vi "Passwort Filter.vi"(9 "Passworte":T1, 10 "aktueller Level":i16) -> (0 "Array Größe":i32, 1 "gefilterte Indexe":i32[](array[numeric]), 2 "Passworte gefiltert":T1)   [LabVIEW 2020, in "Passwort.lvlib"]
uses:
  Passwort.lvlib
  Passwort Array.ctl
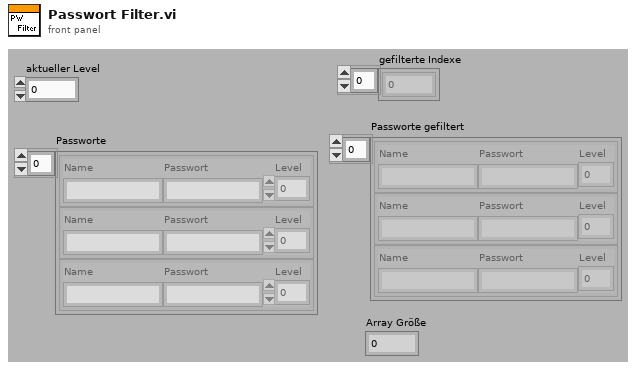
[diagram p1: front panel]
types:
  T1 = typedef "Passwort.lvlib/Passwort Array.ctl" = cluster{"Name":string, "Passwort":string, "Level":i16}[]
  T2 = cluster{"Name":string, "Passwort":string, "Level":i16}
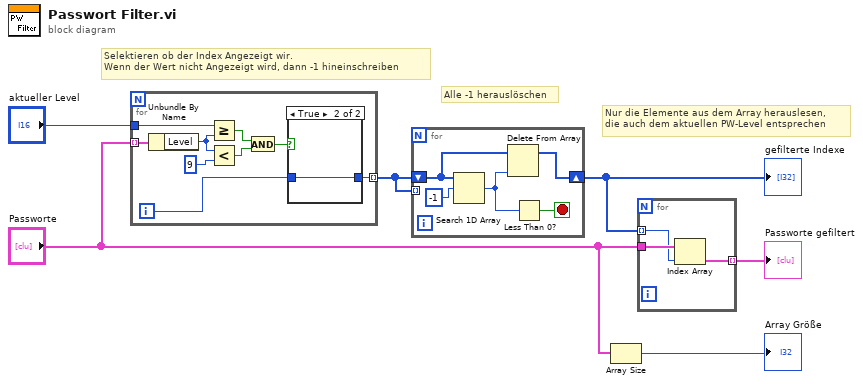
[diagram p0: block diagram]
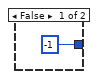
[diagram p2: hidden frame]
diagram:
  # "Nur die Elemente aus dem Array herauslesen, \ndie auch dem aktuellen PW-Level entsprechen"
  # "Alle -1 herauslöschen"
  # "Selektieren ob der Index Angezeigt wir.\nWenn der Wert nicht Angezeigt wird, dann -1 hineinschreiben"
  n1 = for {
    tunnel: "Passworte" -> [w14] mode=indexing
    tunnel: "aktueller Level" -> [w15]
    tunnel: [w12] -> w5 mode=indexing
    i -> [w13]
    n2 = Unbundle By Name(w14) -> ("Level"=w10:i16)
    n3 = Greater Or Equal?(x=w15, y=w10) -> (x >= y?=w8:bool)
    n4 = Less?(x=w10, y=i16 9) -> (x < y?=w11:bool)
    n5 = And(x=w8, y=w11) -> (x .and. y?=w7:bool)
    n6 = case shown="True" w7 {
      tunnel: w13 -> [_ w17]
      tunnel: [-1 w17] -> w12
      frame False {
      }
      frame True {
      }
    }
  }
  n7 = for {
    shift-right: [w20] -> w3
    shift-left: w5 -> [w21]
    tunnel: w5 -> [_] mode=indexing
    stop <- w19 stop-if-true
    n8 = Search 1D Array(1D array=w21, element=-1 ("Element")) -> (index of element=w18:i32)  [unwired: 1 in]
    n9 = Delete From Array(array=w21, index=w18) -> (array with subset deleted=w20:i32[])  [unwired: 1 in, 1 out]
    n10 = Less Than 0?(x=w18) -> (x < 0?=w19:bool)
  }
  "gefilterte Indexe" <- w3
  n11 = Array Size(array="Passworte") -> (size(s)=→"Array Größe":i32)
  n12 = for {
    tunnel: w3 -> [w24] mode=indexing
    tunnel: "Passworte" -> [w25]
    tunnel: [w23] -> w4 mode=indexing
    n13 = Index Array(array=w25, index=w24) -> (element=w23:T2)
  }
  "Passworte gefiltert" <- w4
